vi "Launch Root Model.vi"(8 "error in (no error)":errorcluster, 11 "PublishingViewModel In":refnum<class "PublishingViewModel.lvclass">) -> (0 "error out":errorcluster, 3 "PublishingViewModel Out":refnum<class "PublishingViewModel.lvclass">)   [LabVIEW 2015, in "PublishingViewModel.lvclass"]
doc: "<License>\nCopyright © 2017 Composed Systems, LLC | All rights reserved\nwww.composed.io\n\nAuthor: Ethan Stern <ethan.stern@composed.io>\n\nThis software is provided \"AS IS\" WITHOUT WARRANTIES, either express or implied, AND IS FOR EDUCATIONAL PURPOSES ONLY.\n</License>"
uses:
  PublishingViewModel.lvclass
  <vilib>/ActorFramework/Actor/Actor.lvclass/Actor.ctl
  <vilib>/ActorFramework/Message Enqueuer/Message Enqueuer.lvclass/Message Enqueuer.ctl
  Framework/IViewModel/IViewModel/IViewModel.lvclass/IViewModel.ctl
  Framework/IMediator/PublishRequest/PublishRequest.lvclass/PublishRequest.ctl
  Framework/AbstractMessages/PreAddressedMsg/PreAddressedMsg.lvclass/PreAddressedMsg.ctl
  Framework/IMediator/IMediator Messages/Publish Msg/Publish Msg.lvclass/Publish Msg.ctl
  Framework/IMediator/IMediator Messages/Publish Msg/Send Pre-Addressed Publish.vi
  Framework/IObserver/IObserver/Read Unique ID.vi
  Framework/IMediator/PublishRequest/Pack Publish Request.vi
  <vilib>/ActorFramework/Message Enqueuer/Enqueue.vi
  Framework/AbstractMessages/PreAddressedMsg/Read Return Address.vi
  <vilib>/ActorFramework/Actor/Read Self Enqueuer.vi
  <vilib>/ActorFramework/Message Enqueuer/Init from Existing Queue.vi
  <vilib>/ActorFramework/Message Priority Queue/Priority Enqueue.vi
  Framework/IViewModel/IViewModel/IViewModel.lvclass
  Framework/IMediator/PublishRequest/PublishRequest.lvclass
  <vilib>/ActorFramework/Message Enqueuer/Message Enqueuer.lvclass
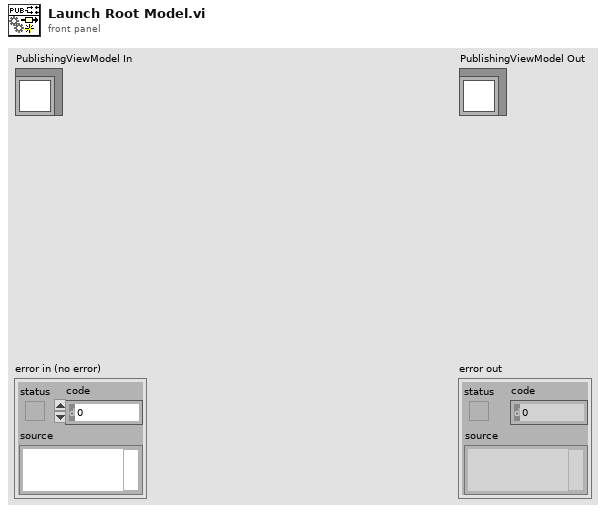
[diagram p1: front panel]
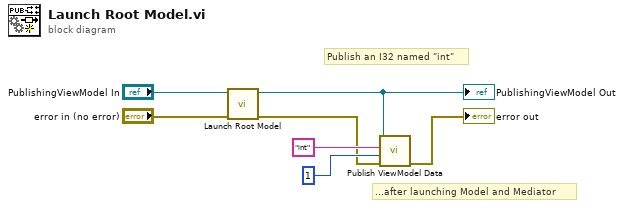
[diagram p0: block diagram]
diagram:
  # "...after launching Model and Mediator"
  # "Publish an I32 named \"int\""
  n1 = call-parent "Launch Root Model.vi"("error in (no error)"="error in (no error)", "IViewModel In"="PublishingViewModel In") -> ("error out"=w3:errorcluster, "IViewModel Out"=w2:refnum<class "PublishingViewModel.lvclass">)  [unwired: 8 in]
  "PublishingViewModel Out" <- w2
  n2 = call "Publish ViewModel Data.vi"("error in (no error)"=w3, "Data to Publish"=1, "Datum Name"="int", "IViewModel In"=w2) -> ("error out"=→"error out":errorcluster)  [unwired: 6 in, 1 out]
